vi "SaveDataFile.vi"(0 "Data Array":dbl[][](array[numeric]), 1 "Temperature":dbl, 2 "Run uninterrupted?":bool, 3 "Humidity":dbl, 5 "no. of arrays":i32, 9 "Actual array lengths":i32, 11 "Error In":errorcluster, 12 "Array Titles":string, 13 "Strip Segment":string, 14 "Arrays format":string) -> (4 "Filename OUT":string, 6 "Pathname OUT":string, 10 "Path + Filename OUT":string, 15 "Error Out":errorcluster)   [LabVIEW 2013]
uses:
  globals/QC_RunInformation.vi
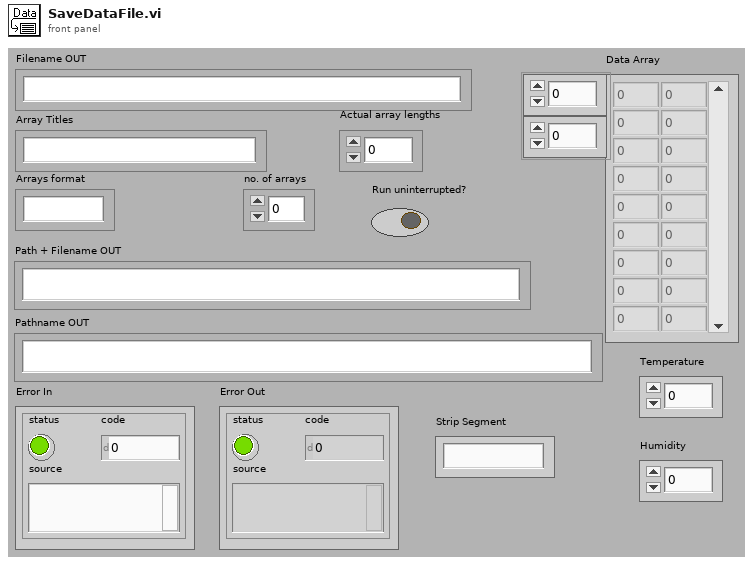
[diagram p1: front panel]
types:
  T1 = enum16{"open", "open or create", "create or replace", "create"}
  T2 = cluster{"Sensor Serial No.:":string, "Wafer:":string, "Batch:":string, "Manufacturer:":string, "Device Category:":string, "Database Serial No.:":string, "Date Initiated:":string, "Time Initiated:":string, "Test":string, "Probeplan used:":string, "End of Run comment:":string, "User:":string, "Vbias SMU":string, "LCR":string, "Test SMU":string, "Test DMM":string}
  T3 = cluster{"Institute":string, "Manufacturers":string[], "Devices":string[], "Serialnumbers Lookup DB":string, "Data directory":string, "Backup & screenshot directory":string, "List of known users":string[], "Measurement switch not used":bool, "Measurement Switch":string, "DUT Switch":string, "Rseries IV [MOhm]":string, "Rshunt IV [MOhm]":string, "Rseries CV [MOhm]":string, "DC blocking Cap [µF]":string, "Rseries LCR [MOhm]":string, "Rseries stability [MOhm]":string, "Rshunt stability [MOhm]":string, "Rseries striptest bias [MOhm]":string, "Rseries strip pinhole [MOhm]":string}
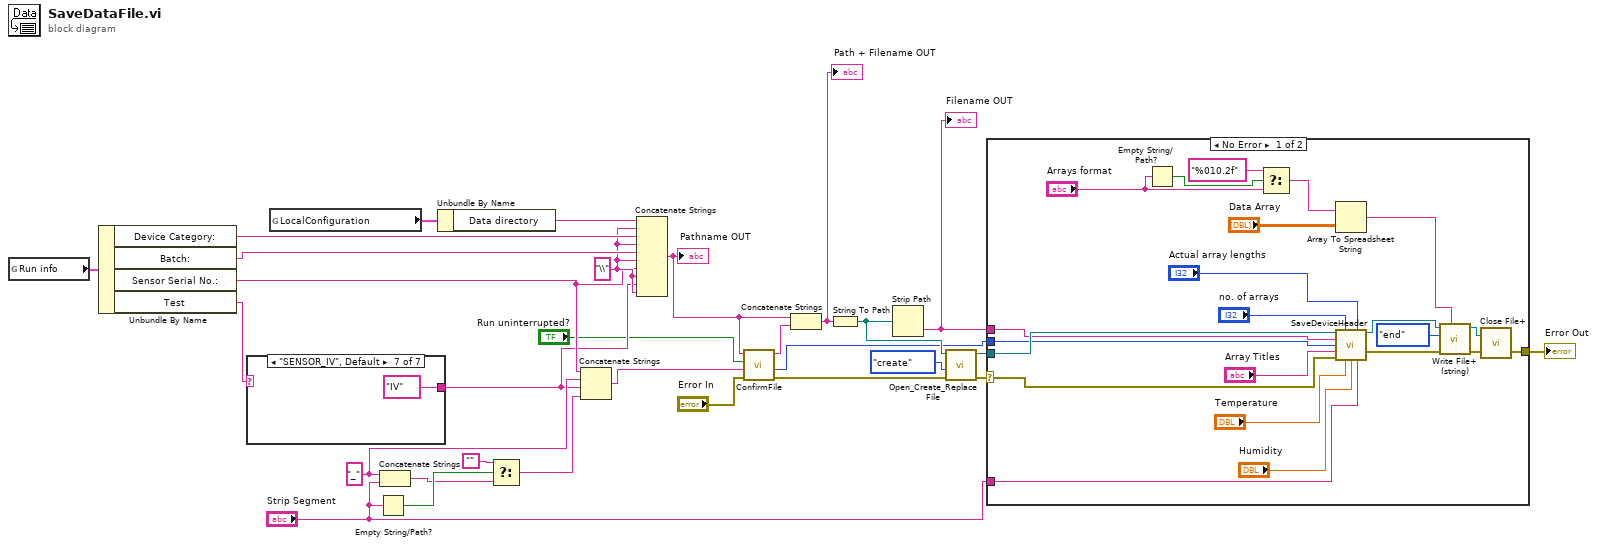
[diagram p0: block diagram]
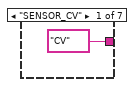
[diagram p2: hidden frame]
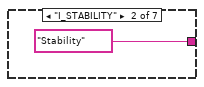
[diagram p3: hidden frame]
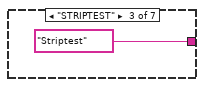
[diagram p4: hidden frame]
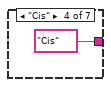
[diagram p5: hidden frame]
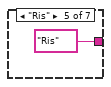
[diagram p6: hidden frame]
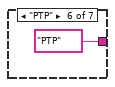
[diagram p7: hidden frame]
diagram:
  w9 = "_"
  w19 = "\\"
  n1 = global read "QC_RunInformation.vi" "Run info"() -> (w28:T2)
  n2 = Unbundle By Name(w28) -> ("Device Category:"=w26:string, "Batch:"=w25:string, "Sensor Serial No.:"=w6:string, "Test"=w3:string)
  n3 = case shown="\"SENSOR_IV\", Default" w3 {
    tunnel: ["CV" ("Test") "Stability" ("Test") "Striptest" ("Test") "Cis" ("Test") "Ris" ("Test") "PTP" ("Test") "IV" ("Test")] -> w2
    frame "SENSOR_CV" {
    }
    frame "I_STABILITY" {
    }
    frame "STRIPTEST" {
    }
    frame "Cis" {
    }
    frame "Ris" {
    }
    frame "PTP" {
    }
    frame "SENSOR_IV", Default {
    }
  }
  n4 = global read "QC_RunInformation.vi" "LocalConfiguration"() -> (w29:T3)
  n5 = Empty String/Path?(string/path="Strip Segment") -> (empty?=w11:bool)
  n6 = Concatenate Strings(w9, "Strip Segment") -> (w7:string)
  n7 = Unbundle By Name(w29) -> ("Data directory"=w27:string)
  n8 = Select(t="", s=w11, f=w7) -> (s? t:f=w8:string)
  n9 = Concatenate Strings(w6, w9, w2, w8) -> (w18:string)
  n10 = Concatenate Strings(w27, w19, w26, w19, w25, w19, w6, w19, w2, w19) -> (w14:string)
  "Pathname OUT" <- w14
  n11 = call "ConfirmFile.vi"("Error In"="Error In", "Filename IN"=w18, "Run uninterrupted?"="Run uninterrupted?", "Pathname IN"=w14) -> ("Error Out"=w15:errorcluster, "Run Number"=w5:i32, "Filename:"=w13:string)  [unwired: 1 in]
  n12 = Concatenate Strings(w14, w13) -> (w12:string)
  "Path + Filename OUT" <- w12
  n13 = String To Path(string=w12) -> (path=w21:path)
  n14 = Strip Path(path=w21) -> (name=w22:string)  [unwired: 1 out]
  "Filename OUT" <- w22
  n15 = call <vilib>:"Open_Create_Replace File.vi"("error in (no error)"=w15, "function (open:0)"=T1."create", "file path"=w21) -> ("error out"=w20:errorcluster, "refnum"=w23:refnum<file>)  [unwired: 5 in, 2 out]
  n16 = case shown="No Error" w20 {
    selector: w20 -> [w58 w59]
    tunnel: w23 -> [w47 _]
    tunnel: w22 -> [w46 _]
    tunnel: [w42 w59] -> w17
    tunnel: w5 -> [w38 _]
    tunnel: "Strip Segment" -> [w37 _]
    frame No Error {
      n17 = Empty String/Path?(string/path="Arrays format") -> (empty?=w55:bool)
      n18 = Select(t="%010.2f", s=w55, f="Arrays format") -> (s? t:f=w53:string)
      n19 = Array To Spreadsheet String(array="Data Array", 3:w53) -> (spreadsheet string=w52:string)  [unwired: 1 in]
      n20 = call "SaveDeviceHeader.vi"("File Refnum in"=w47, "no. of arrays"="no. of arrays", "Array Lengths"="Actual array lengths", "Filename"=w46, "Run Number"=w38, "Array Titles"="Array Titles", "error in (no error)"=w58, "Temperature"="Temperature", "Humidity"="Humidity", "Strip Segment"=w37) -> ("File Refnum out"=w48:refnum<file>, "error out"=w39:errorcluster)  [unwired: 3 in, 1 out]
      n21 = call <vilib>:"Write File+ (string).vi"("string"=w52, "error in (no error)"=w39, "pos mode (rel. to end:1)"=enum16{"start", "end", "current"}."end", "refnum"=w48) -> ("error out"=w51:errorcluster, "dup refnum"=w49:refnum<file>)  [unwired: 3 in, 1 out]
      n22 = call <vilib>:"Close File+.vi"("error in (no error)"=w51, "refnum"=w49) -> ("error out"=w42:errorcluster)  [unwired: 3 in, 2 out]
    }
    frame Error {
    }
  }
  "Error Out" <- w17
